vi "Initialization VI.vi"(8 "error in (no error)":errorcluster, 10 "Custom XML":string, 11 "Device Item Ref in":T1 format="%.0x") -> (0 "error out":errorcluster, 3 "Device Item Ref out":T1 format="%.0x")   [LabVIEW 2015, in "SLSC Module Template System Explorer.lvlib"]
uses:
  SLSC Module Template System Explorer.lvlib
  <vilib>/NI Veristand/Custom Device API/Custom Device Item Ref.ctl
  Shared/Constants.vi
  <vilib>/NI Veristand/Custom Device API/Set Item Property (String).vi
  <vilib>/NI Veristand/Custom Device API/Set Item Property (I32).vi
  <vilib>/NI Veristand/Custom Device API/Custom Device API.lvlib
  Shared/SLSC Module Template Shared.lvlib
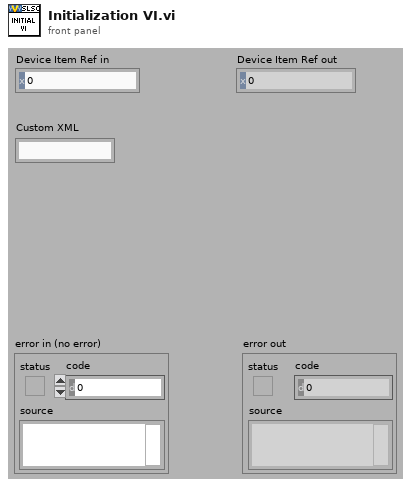
[diagram p1: front panel]
types:
  T1 = typedef "Custom Device API.lvlib/Custom Device Item Ref.ctl" = u64
  T2 = typedef "Custom Device API.lvlib/Custom Device Channel.ctl" = cluster{"Type":T3, "Units":string, "Default Value":dbl, "Faultable":bool, "Scalable":bool}
  T3 = typedef "Custom Device API.lvlib/Custom Device Channel Type.ctl" = enum16{"Input", "Output"}
  T4 = cluster{"Channel Name":string, "SLSC Name":string, "Channel":T2}[]
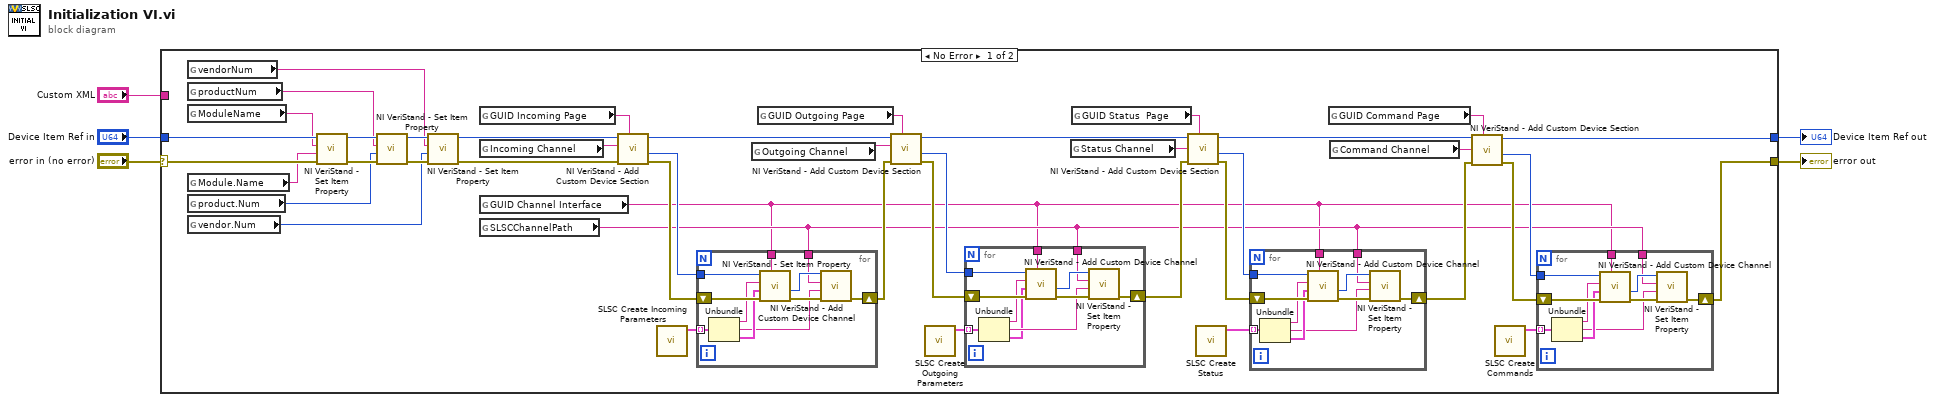
[diagram p0: block diagram]
diagram:
  n1 = case shown="No Error" "error in (no error)" {
    selector: "error in (no error)" -> [w36 w95]
    tunnel: [w11 w95] -> w5
    tunnel: [w10 w94] -> w3
    tunnel: "Device Item Ref in" -> [w39 w94]
    tunnel: "Custom XML" -> [_ _]
    frame No Error {
      n2 = global read "Constants.vi" "vendorNum"() -> (w33:string)
      n3 = global read "Constants.vi" "productNum"() -> (w34:string)
      n4 = global read "Constants.vi" "ModuleName"() -> (w35:string)
      n5 = global read "Constants.vi" "Module.Name"() -> (w32:string)
      n6 = global read "Constants.vi" "product.Num"() -> (w31:i32)
      n7 = global read "Constants.vi" "vendor.Num"() -> (w30:i32)
      n8 = call-poly <vilib>:"NI VeriStand - Set Item Property.vi"("error in (no error)"=w36, "Value"=w32, "Property Name"=w35, "Item Ref in"=w39) -> ("error out"=w41:errorcluster, "Item Ref out"=w43:T1)  [unwired: 5 in, 1 out]
      n9 = call-poly <vilib>:"NI VeriStand - Set Item Property.vi"("error in (no error)"=w41, "Value"=w31, "Property Name"=w34, "Item Ref in"=w43) -> ("error out"=w40:errorcluster, "Item Ref out"=w42:T1)  [unwired: 5 in, 1 out]
      n10 = call-poly <vilib>:"NI VeriStand - Set Item Property.vi"("error in (no error)"=w40, "Value"=w30, "Property Name"=w33, "Item Ref in"=w42) -> ("error out"=w37:errorcluster, "Item Ref out"=w38:T1)  [unwired: 5 in, 1 out]
      n11 = global read "Constants.vi" "GUID Incoming Page"() -> (w22:string)
      n12 = global read "Constants.vi" "Incoming Channel"() -> (w29:string)
      n13 = global read "Constants.vi" "GUID Channel Interface"() -> (w12:string)
      n14 = global read "Constants.vi" "SLSCChannelPath"() -> (w13:string)
      n15 = call <vilib>:"NI VeriStand - Add Custom Device Section.vi"("GUID (Default Section)"=w22, "error in (no error)"=w37, "Section Name"=w29, "Parent Ref in"=w38) -> ("error out"=w49:errorcluster, "Section Ptr"=w48:T1, "Parent Ref out"=w47:T1)  [unwired: 4 in, 1 out]
      n16 = call "SLSC Create Incoming Parameters.vi"() -> ("Outgoing configuration"=w8:T4)  [unwired: 11 in]
      n17 = for {
        tunnel: w48 -> [w88]
        shift-right: [w91] -> w46
        shift-left: w49 -> [w87]
        tunnel: w13 -> [w90]
        tunnel: w12 -> [w89]
        tunnel: w8 -> [w86] mode=indexing
        n18 = Unbundle(w86) -> ("Channel Name"=w85:string, "SLSC Name"=w83:string, "Channel"=w84:T2)
        n19 = call <vilib>:"NI VeriStand - Add Custom Device Channel.vi"("GUID (Default Channel)"=w89, "error in (no error)"=w87, "Channel"=w84, "Channel Name"=w85, "Parent Ref in"=w88) -> ("error out"=w92:errorcluster, "Channel Ref"=w93:T1)  [unwired: 3 in, 2 out]
        n20 = call-poly <vilib>:"NI VeriStand - Set Item Property.vi"("error in (no error)"=w92, "Value"=w83, "Property Name"=w90, "Item Ref in"=w93) -> ("error out"=w91:errorcluster)  [unwired: 5 in, 2 out]
      }
      n21 = global read "Constants.vi" "Outgoing Channel"() -> (w28:string)
      n22 = global read "Constants.vi" "GUID Outgoing Page"() -> (w21:string)
      n23 = call <vilib>:"NI VeriStand - Add Custom Device Section.vi"("GUID (Default Section)"=w21, "error in (no error)"=w46, "Section Name"=w28, "Parent Ref in"=w47) -> ("error out"=w45:errorcluster, "Section Ptr"=w44:T1, "Parent Ref out"=w27:T1)  [unwired: 4 in, 1 out]
      n24 = call "SLSC Create Outgoing Parameters.vi"() -> ("Outgoing configuration"=w9:T4)  [unwired: 11 in]
      n25 = for {
        tunnel: w44 -> [w77]
        shift-right: [w80] -> w25
        shift-left: w45 -> [w76]
        tunnel: w13 -> [w79]
        tunnel: w12 -> [w78]
        tunnel: w9 -> [w75] mode=indexing
        n26 = Unbundle(w75) -> ("Channel Name"=w74:string, "SLSC Name"=w73:string, "Channel"=w72:T2)
        n27 = call <vilib>:"NI VeriStand - Add Custom Device Channel.vi"("GUID (Default Channel)"=w78, "error in (no error)"=w76, "Channel"=w72, "Channel Name"=w74, "Parent Ref in"=w77) -> ("error out"=w81:errorcluster, "Channel Ref"=w82:T1)  [unwired: 3 in, 2 out]
        n28 = call-poly <vilib>:"NI VeriStand - Set Item Property.vi"("error in (no error)"=w81, "Value"=w73, "Property Name"=w79, "Item Ref in"=w82) -> ("error out"=w80:errorcluster)  [unwired: 5 in, 2 out]
      }
      n29 = global read "Constants.vi" "Status Channel"() -> (w26:string)
      n30 = global read "Constants.vi" "GUID Status  Page"() -> (w20:string)
      n31 = call <vilib>:"NI VeriStand - Add Custom Device Section.vi"("GUID (Default Section)"=w20, "error in (no error)"=w25, "Section Name"=w26, "Parent Ref in"=w27) -> ("error out"=w24:errorcluster, "Section Ptr"=w23:T1, "Parent Ref out"=w16:T1)  [unwired: 4 in, 1 out]
      n32 = call "SLSC Create Status.vi"() -> ("Outgoing configuration"=w6:T4)  [unwired: 11 in]
      n33 = for {
        tunnel: w23 -> [w66]
        shift-right: [w69] -> w17
        shift-left: w24 -> [w65]
        tunnel: w13 -> [w68]
        tunnel: w12 -> [w67]
        tunnel: w6 -> [w64] mode=indexing
        n34 = Unbundle(w64) -> ("Channel Name"=w63:string, "SLSC Name"=w61:string, "Channel"=w62:T2)
        n35 = call <vilib>:"NI VeriStand - Add Custom Device Channel.vi"("GUID (Default Channel)"=w67, "error in (no error)"=w65, "Channel"=w62, "Channel Name"=w63, "Parent Ref in"=w66) -> ("error out"=w70:errorcluster, "Channel Ref"=w71:T1)  [unwired: 3 in, 2 out]
        n36 = call-poly <vilib>:"NI VeriStand - Set Item Property.vi"("error in (no error)"=w70, "Value"=w61, "Property Name"=w68, "Item Ref in"=w71) -> ("error out"=w69:errorcluster)  [unwired: 5 in, 2 out]
      }
      n37 = global read "Constants.vi" "GUID Command Page"() -> (w15:string)
      n38 = global read "Constants.vi" "Command Channel"() -> (w14:string)
      n39 = call <vilib>:"NI VeriStand - Add Custom Device Section.vi"("GUID (Default Section)"=w15, "error in (no error)"=w17, "Section Name"=w14, "Parent Ref in"=w16) -> ("error out"=w18:errorcluster, "Section Ptr"=w19:T1, "Parent Ref out"=w10:T1)  [unwired: 4 in, 1 out]
      n40 = call "SLSC Create Commands.vi"() -> ("Outgoing configuration"=w7:T4)  [unwired: 11 in]
      n41 = for {
        tunnel: w19 -> [w55]
        shift-right: [w58] -> w11
        shift-left: w18 -> [w54]
        tunnel: w13 -> [w57]
        tunnel: w12 -> [w56]
        tunnel: w7 -> [w53] mode=indexing
        n42 = Unbundle(w53) -> ("Channel Name"=w52:string, "SLSC Name"=w50:string, "Channel"=w51:T2)
        n43 = call <vilib>:"NI VeriStand - Add Custom Device Channel.vi"("GUID (Default Channel)"=w56, "error in (no error)"=w54, "Channel"=w51, "Channel Name"=w52, "Parent Ref in"=w55) -> ("error out"=w59:errorcluster, "Channel Ref"=w60:T1)  [unwired: 3 in, 2 out]
        n44 = call-poly <vilib>:"NI VeriStand - Set Item Property.vi"("error in (no error)"=w59, "Value"=w50, "Property Name"=w57, "Item Ref in"=w60) -> ("error out"=w58:errorcluster)  [unwired: 5 in, 2 out]
      }
    }
    frame Error {
    }
  }
  "error out" <- w5
  "Device Item Ref out" <- w3
